vi "Trans-FPGA.vi"() -> ()   [LabVIEW 2016]
uses:
  Gate Valve Readback.ctl
  Faraday Cup Readback.ctl
  <vilib>/LabVIEW Targets/FPGA/cRIO/shared/nicrio_ModuleControls/nicrio_cRIO-9871_DataBitsEnum.ctl
  <vilib>/LabVIEW Targets/FPGA/cRIO/shared/nicrio_ModuleControls/nicrio_cRIO-9871_BaudRateEnum.ctl
  <vilib>/LabVIEW Targets/FPGA/cRIO/shared/nicrio_ModuleControls/nicrio_cRIO-9871_ParityEnum.ctl
  <vilib>/LabVIEW Targets/FPGA/cRIO/shared/nicrio_ModuleControls/nicrio_cRIO-9871_StopBitsEnum.ctl
  <vilib>/Platform/TimedLoop/XDataNode/timing_clust.ctl
  <vilib>/Platform/TimedLoop/XDataNode/nitl_modes.ctl
  <vilib>/Platform/TimedLoop/XDataNode/wakeup.ctl
  <vilib>/rvi/FXPMathLib/basic elements/FxpIntAccumulator/subVIs/nifxpmath_IntAccumulator_SimConfig.ctl
  <vilib>/rvi/Emulation/niFpgaGetClockAttributes.vi
  <vilib>/rvi/Emulation/niFpgaSctlEmulationGetInTimedLoop.vi
  <vilib>/rvi/Emulation/niFpgaEmulationReportErrorSimple.vi
  <vilib>/rvi/eio/common/nirviEmuTemplateMethod_errors.vi
  <vilib>/rvi/Emulation/niFpgaCriticalErrorInLSC.vi
  <vilib>/rvi/Analysis/common/codeGenErrors/XNode/niFpgaXNodeCodeGenErrorHandle.vi
  <vilib>/rvi/FXPMathLib/basic elements/FxpIntAccumulator/simVIs/DllFxpIntAccumulator_sub.vi
  <vilib>/rvi/eio/common/nirviEmuTemplatePropertySet_errors.vi
  <vilib>/eio/EIONode/EIONode.xnode
  <vilib>/rvi/Analysis/measure/dc-rms/XNode/niFpgaDC-RMS.xnode
  <vilib>/Platform/TimedLoop/XDataNode/XDataNode.xnode
  <vilib>/rvi/FXPMathLib/basic elements/FxpIntAccumulator/XNode/nifxpmath_IntAccumulator.xnode
  <vilib>/rvi/FXPMathLib/FxpMul/XNode/nifxpmath_Multiplier.xnode
  <vilib>/eio/EIOPropertyNode/EIOPropertyNode.xnode
  <vilib>/eio/EIOMethodNode/EIOMethodNode.xnode
  <vilib>/Platform/TimedLoop/XDataNode/XDNodeRunTimeDep.lvlib
  <vilib>/rvi/FXPMathLib/sim/FxpSim.dll
  <vilib>/rvi/eio/common/nirviEmuTemplatePropertyGet_errors.vi
  <vilib>/rvi/eio/common/nirviEmuTemplatePropertyGet_noerrors.vi
  <vilib>/rvi/eio/common/nirviEmuTemplatePropertySet_noerrors.vi
panel:
  in  "Analzyer Image FC Actuator":bool
  out "Analzyer Image FC Position":T1
  in  "Switch Object Interlock Bypass":bool
  in  "Analyzer Image Interlock Bypass":bool
  in  "Turbo 1 GV Actuator":bool
  in  "Beamline GV Actuator":bool
  in  "Turbo 2 GV Actuator":bool
  out "Analyzer Image Vac Interlock":bool
  out "Switch Object Vac Interlock":bool
  out "GV Interlock loop error":errorcluster
  out "Turbo 1 GV Status":T2
  out "Turbo 2 GV Status":T2
  out "Beamline GV Status":T2
  out "Actuator-Sensor Loop error":errorcluster
  in  "HV Enable":bool[](array[boolean])=[FALSE, FALSE, FALSE, FALSE, FALSE, FALSE]
  out "Switch Object Vacuum Error":errorcluster
  out "Analyze Image Vacuum Error":errorcluster
  out "Switch PS error":errorcluster
  out "ExB PS error":errorcluster
  out "Analyzer PS error":errorcluster
  out "9264 error":errorcluster
  out "9205 error":errorcluster
  in  "RT error":bool
  in  "switch mag ps set":u8[](array[numeric])=[0, 0, 0, 0, 0, 0, 0, 0, 0, 0]
  out "Switch mag data":u8
  out "Switch Mag Hall Probe Timed out":bool
  out "switch mag field":u8[](array[numeric])
  out "Switch Hall Probe error":errorcluster
  in  "trans ExB mag ps set":u8[](array[numeric])=[0, 0, 0, 0, 0, 0, 0, 0, 0, 0]
  in  "analyzer mag ps set":u8[](array[numeric])=[0, 0, 0, 0, 0, 0, 0, 0, 0, 0]
  out "analyzer mag data":u8
  out "Timed Out":bool
  out "analyzer mag field":u8[](array[numeric])
  out "Analyzer Hall Probe error":errorcluster
  out "Ion gauge 4":u8[](array[numeric])
  out "Convectron 4":u8[](array[numeric])
  out "Convectron 3":u8[](array[numeric])
  out "Ion gauge 3":u8[](array[numeric])
  out "Ion gauge 2":u8[](array[numeric])
  out "Convectron 2":u8[](array[numeric])
  out "Convectron 1":u8[](array[numeric])
  out "Ion gauge 1":u8[](array[numeric])
  in  "HV Set":fxp<+/-,26,5>[](array[numeric])=[0.0, 0.0, 0.0, 0.0, 0.0, 0.0] format="%.23g"
  out "HV monitor":fxp<+/-,26,5>[](array[numeric]) format="%.23g"
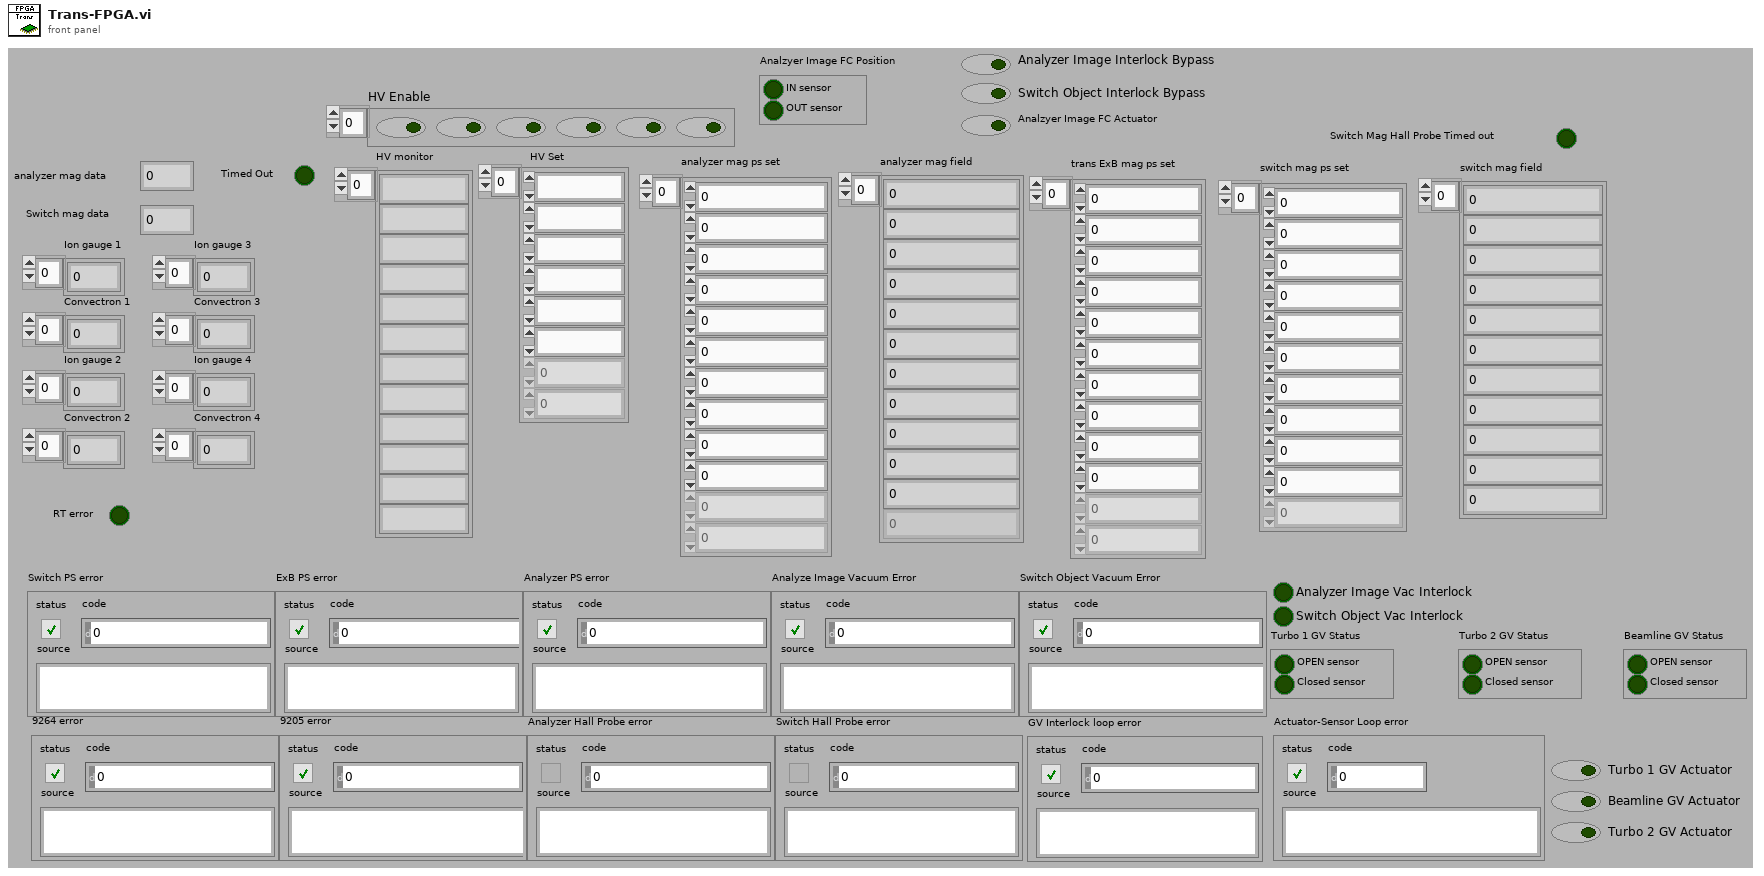
[diagram p1: front panel]
types:
  T1 = typedef "Faraday Cup Readback.ctl" = cluster{"IN sensor":bool, "OUT sensor":bool}
  T2 = typedef "Gate Valve Readback.ctl" = cluster{"OPEN sensor":bool, "Closed sensor":bool}
  T3 = typedef "nicrio_cRIO-9871_BaudRateEnum.ctl" = enum16{"75 bps", "110 bps", "134 bps", "150 bps", "300 bps", "600 bps", "1200 bps", "1800 bps", "2400 bps", "4800 bps", "7200 bps", "9600 bps", "14.4 kbps", "19.2 kbps", "28.8 kbps", "38.4 kbps", "57.6 kbps", "115.2 kbps", "230.4 kbps", "460.8 kbps", "921.6 kbps"}
  T4 = typedef "nicrio_cRIO-9871_DataBitsEnum.ctl" = enum8{"5", "6", "7", "8"}
  T5 = typedef "nicrio_cRIO-9871_StopBitsEnum.ctl" = enum8{"1", "1.5", "2"}
  T6 = typedef "nicrio_cRIO-9871_ParityEnum.ctl" = enum8{"None", "Odd", "Even", "Mark", "Space"}
  T7 = typedef "XDNodeRunTimeDep.lvlib/timing_clust.ctl" = cluster{"Expected End [f-1]":u64, "Actual End [f-1]":u64, "Finished Late? [f-1]":bool, "Expected End [i-1]":u64, "Actual End [i-1]":u64, "Finished Late? [i-1]":bool, "Expected Start [i]":u64, "Actual Start [i]":u64, "Expected Start [f]":u64, "Actual Start [f]":u64, "Source Name":string, "Structure Name":string, "Period":i64, "Deadline":i64, "Offset":i64, "Start":i64, "Priority":i32, "Timeout":i32, "Mode":T8, "Wakeup Reason":T9, "Error":errorcluster, "Source Type":string, "Secondary Source Type":string, "Global End Time":u64, "Global Start Time":u64, "Frame Duration":u64, "Iteration Duration":u64, "Assigned CPU":i32, "I/O Scan Engine Mode":u32}
  T8 = typedef "XDNodeRunTimeDep.lvlib/nitl_modes.ctl" = enum32{"No Change", "Process missed periods, maintain original phase", "Discard missed periods, maintain original phase", "Process missed periods, ignore original phase", "Discard missed periods, ignore original phase"}
  T9 = typedef "XDNodeRunTimeDep.lvlib/wakeup.ctl" = enum32{"Normal", "Aborted", "Asynchronous wakeup", "Timing source error", "Timed loop error", "Timeout"}
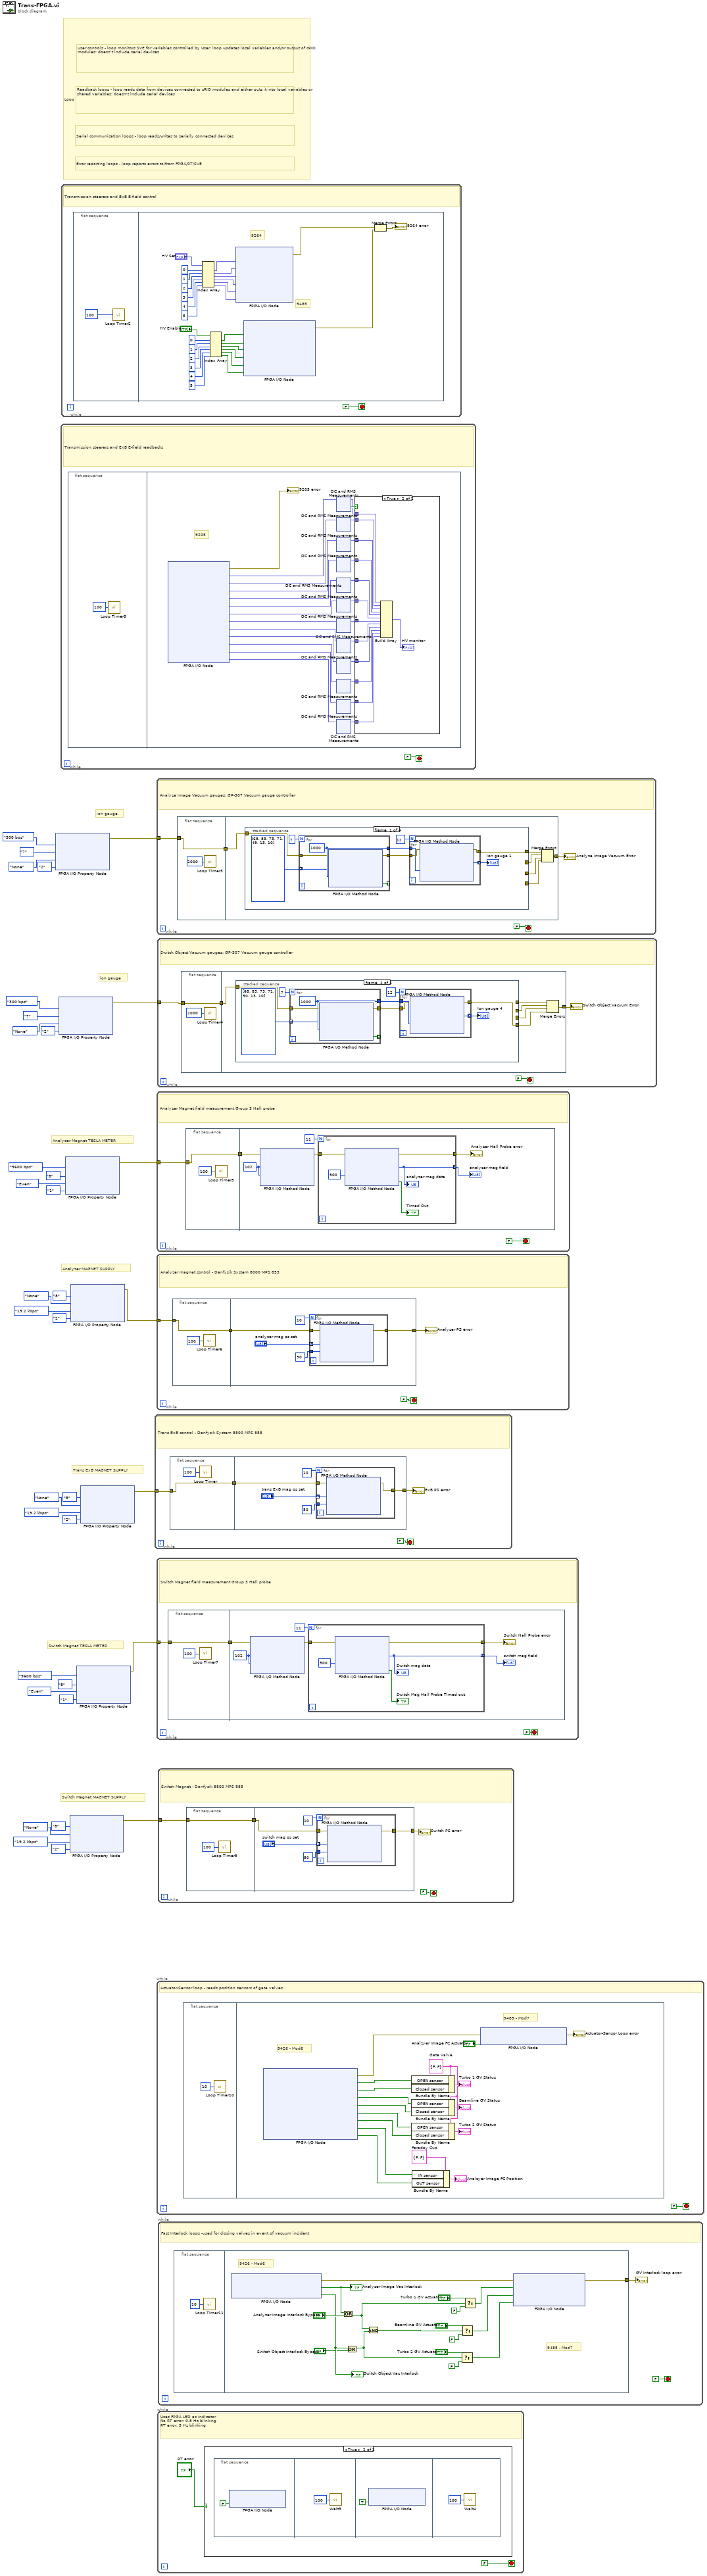
[diagram p0: block diagram]
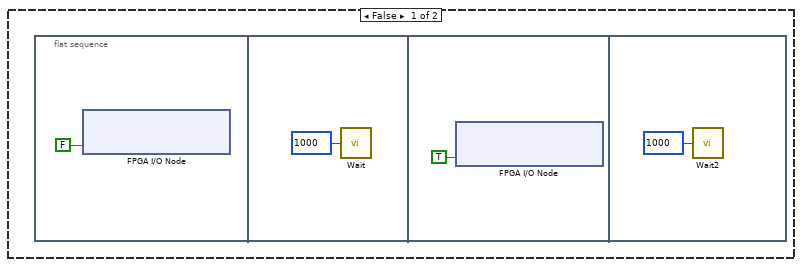
[diagram p2: hidden frame]
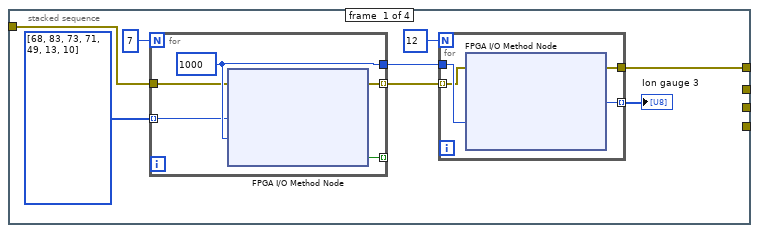
[diagram p4: hidden frame]
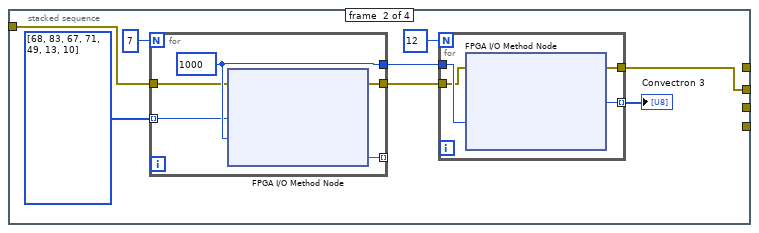
[diagram p5: hidden frame]
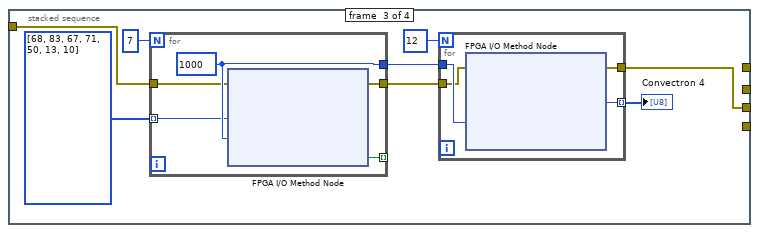
[diagram p6: hidden frame]
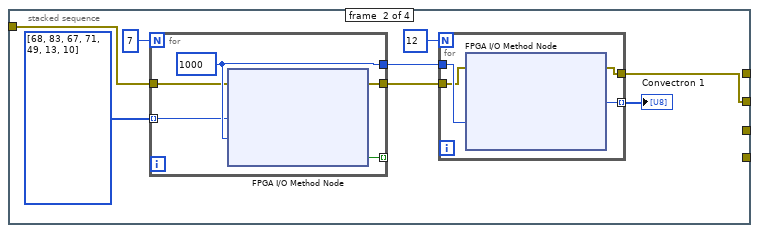
[diagram p7: hidden frame]
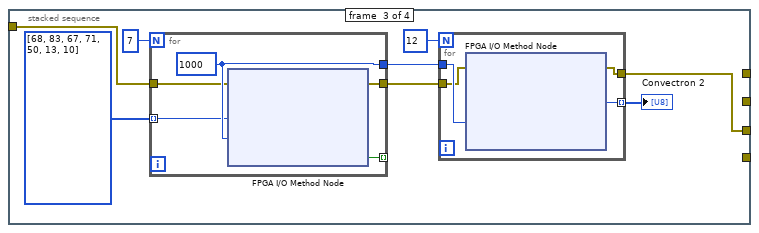
[diagram p8: hidden frame]
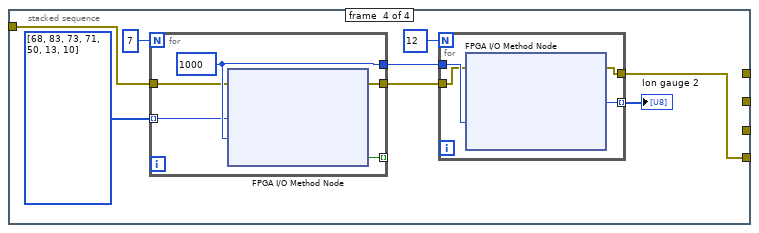
[diagram p9: hidden frame]
diagram:
  # "Error reporting loops - loop reports errors to/from FPGA/RT/SVE"
  # "Serial communication loops - loop reads/writes to serially connected devices"
  # "Readback loops - loop reads data from devices connected to cRIO modules and either puts it into local variables or shared variables; doesn't include serial devices"
  # "User controls - loop monitors SVE for variables controlled by User; loop updates local variables and/or output of cRIO modules; doesn't include serial devices"
  # "Loop legend - loops are color coded by responsibility"
  # "Switch Magnet TESLA METER"
  # "Switch Magnet MAGNET SUPPLY"
  # "Trans ExB MAGNET SUPPLY"
  # "ion gauge"
  # "Analyzer MAGNET SUPPLY"
  # "Analyzer Magnet TESLA METER"
  # "ion gauge"
  n1 = xnode "FPGA I/O Property Node"("Baud Rate"=nicrio_cRIO-9871_BaudRateEnum."300 bps", "Data Bits"=nicrio_cRIO-9871_DataBitsEnum."7", "Parity"=nicrio_cRIO-9871_ParityEnum."None", "Stop Bits"=nicrio_cRIO-9871_StopBitsEnum."2") -> ("error out"=w6:errorcluster)  [unwired: 2 in, 1 out]
  n2 = xnode "FPGA I/O Property Node"("Baud Rate"=nicrio_cRIO-9871_BaudRateEnum."300 bps", "Data Bits"=nicrio_cRIO-9871_DataBitsEnum."7", "Parity"=nicrio_cRIO-9871_ParityEnum."None", "Stop Bits"=nicrio_cRIO-9871_StopBitsEnum."2") -> ("error out"=w7:errorcluster)  [unwired: 2 in, 1 out]
  n3 = while {
    stop <- FALSE stop-if-true
    # "Transmission steerers and ExB E-field readbacks"
    n4 = flat-sequence {
      frame #0 {
        n5 = call "Loop Timer8"("Count(mSec)"=u32 100 ("Count(Ticks)")) -> ()  [unwired: 1 out]
      }
      frame #1 {
        # "9205"
        n6 = xnode "FPGA I/O Node"() -> ("error out"=→"9205 error":errorcluster, "X-steerer+ V read"=w62:fxp<+/-,26,5>, "X-steerer+ I read"=w60:fxp<+/-,26,5>, "X-steerer- V read"=w58:fxp<+/-,26,5>, "X-steerer- I read"=w56:fxp<+/-,26,5>, "Y-steerer+ V read"=w54:fxp<+/-,26,5>, "Y-steerer+ I read"=w52:fxp<+/-,26,5>, "Y-steerer- V read"=w50:fxp<+/-,26,5>, "Y-steerer- I read"=w48:fxp<+/-,26,5>, "ExB+ V read"=w46:fxp<+/-,26,5>, "ExB+ I read"=w44:fxp<+/-,26,5>, "ExB- V read"=w42:fxp<+/-,26,5>, "ExB- I read"=w40:fxp<+/-,26,5>)  [unwired: 13 in, 12 out]
        n7 = xnode "DC and RMS Measurements"("input data"=w62) -> ("DC"=w61:fxp<+/-,26,5>, "output valid"=w63:bool)  [unwired: 1 in]
        n8 = xnode "DC and RMS Measurements"("input data"=w60) -> ("DC"=w59:fxp<+/-,26,5>)  [unwired: 1 in, 1 out]
        n9 = xnode "DC and RMS Measurements"("input data"=w58) -> ("DC"=w57:fxp<+/-,26,5>)  [unwired: 1 in, 1 out]
        n10 = xnode "DC and RMS Measurements"("input data"=w56) -> ("DC"=w55:fxp<+/-,26,5>)  [unwired: 1 in, 1 out]
        n11 = xnode "DC and RMS Measurements"("input data"=w54) -> ("DC"=w53:fxp<+/-,26,5>)  [unwired: 1 in, 1 out]
        n12 = xnode "DC and RMS Measurements"("input data"=w52) -> ("DC"=w51:fxp<+/-,26,5>)  [unwired: 1 in, 1 out]
        n13 = xnode "DC and RMS Measurements"("input data"=w50) -> ("DC"=w49:fxp<+/-,26,5>)  [unwired: 1 in, 1 out]
        n14 = xnode "DC and RMS Measurements"("input data"=w48) -> ("DC"=w47:fxp<+/-,26,5>)  [unwired: 1 in, 1 out]
        n15 = xnode "DC and RMS Measurements"("input data"=w46) -> ("DC"=w45:fxp<+/-,26,5>)  [unwired: 1 in, 1 out]
        n16 = xnode "DC and RMS Measurements"("input data"=w44) -> ("DC"=w43:fxp<+/-,26,5>)  [unwired: 1 in, 1 out]
        n17 = xnode "DC and RMS Measurements"("input data"=w42) -> ("DC"=w41:fxp<+/-,26,5>)  [unwired: 1 in, 1 out]
        n18 = xnode "DC and RMS Measurements"("input data"=w40) -> ("DC"=w39:fxp<+/-,26,5>)  [unwired: 1 in, 1 out]
        n19 = case shown="True" w63 {
          tunnel: w61 -> [_ w76]
          tunnel: w59 -> [_ w75]
          tunnel: w57 -> [_ w74]
          tunnel: w55 -> [_ w73]
          tunnel: w53 -> [_ w72]
          tunnel: w51 -> [_ w71]
          tunnel: w49 -> [_ w70]
          tunnel: w47 -> [_ w69]
          tunnel: w45 -> [_ w68]
          tunnel: w43 -> [_ w67]
          tunnel: w41 -> [_ w66]
          tunnel: w39 -> [_ w65]
          frame False {
          }
          frame True {
            n20 = Build Array(w76, w75, w74, w73, w72, w71, w70, w69, w68, w67, w66, w65) -> (→"HV monitor":fxp<+/-,26,5>[])
          }
        }
      }
    }
  }
  n21 = while {
    stop <- FALSE stop-if-true
    # "Transmission steerers and ExB E-field control"
    n22 = flat-sequence {
      frame #0 {
        n23 = call "Loop Timer2"("Count(mSec)"=u32 100 ("Count(Ticks)")) -> ()  [unwired: 1 out]
      }
      frame #1 {
        # "9485"
        # "9264"
        n24 = Index Array(array="HV Set", index #1=0 ("index"), index #2=1 ("index"), index #3=2 ("index"), index #4=3 ("index"), index #5=4 ("index"), index #6=5 ("index")) -> (element #1=w1062:fxp<+/-,26,5>, element #2=w1061:fxp<+/-,26,5>, element #3=w1060:fxp<+/-,26,5>, element #4=w1055:fxp<+/-,26,5>, element #5=w1057:fxp<+/-,26,5>, element #6=w1056:fxp<+/-,26,5>)
        n25 = Index Array(array="HV Enable", index #1=0 ("index"), index #2=1 ("index"), index #3=2 ("index"), index #4=3 ("index"), index #5=4 ("index"), index #6=5 ("index")) -> (element #1=w1045:bool, element #2=w1044:bool, element #3=w1043:bool, element #4=w1042:bool, element #5=w1041:bool, element #6=w1040:bool)
        n26 = xnode "FPGA I/O Node"("X-steerer+ V set"=w1062, "X-steerer- V set"=w1061, "Y-steerer+ V set"=w1060, "Y-steerer- V set"=w1055, "ExB+ V set"=w1057, "ExB- V set"=w1056) -> ("error out"=w1054:errorcluster)  [unwired: 7 in, 6 out]
        n27 = xnode "FPGA I/O Node"("X-Steerer+ HV Enable"=w1045, "X-Steerer- HV Enable"=w1044, "Y-Steerer+ HV Enable"=w1043, "Y-Steerer- HV Enable"=w1042, "ExB+ HV Enable"=w1041, "ExB- HV Enable"=w1040) -> ("error out"=w1052:errorcluster)  [unwired: 7 in, 6 out]
        n28 = Merge Errors(w1054, w1052) -> (→"9264 error":errorcluster)
      }
    }
  }
  n29 = xnode "FPGA I/O Property Node"("Baud Rate"=nicrio_cRIO-9871_BaudRateEnum."9600 bps", "Data Bits"=nicrio_cRIO-9871_DataBitsEnum."8", "Parity"=nicrio_cRIO-9871_ParityEnum."Even", "Stop Bits"=nicrio_cRIO-9871_StopBitsEnum."1") -> ("error out"=w8:errorcluster)  [unwired: 2 in, 1 out]
  n30 = xnode "FPGA I/O Property Node"("Data Bits"=nicrio_cRIO-9871_DataBitsEnum."8", "Parity"=nicrio_cRIO-9871_ParityEnum."None", "Baud Rate"=nicrio_cRIO-9871_BaudRateEnum."19.2 kbps", "Stop Bits"=nicrio_cRIO-9871_StopBitsEnum."2") -> ("error out"=w10:errorcluster)  [unwired: 2 in, 1 out]
  n31 = xnode "FPGA I/O Property Node"("Data Bits"=nicrio_cRIO-9871_DataBitsEnum."8", "Parity"=nicrio_cRIO-9871_ParityEnum."None", "Baud Rate"=nicrio_cRIO-9871_BaudRateEnum."19.2 kbps", "Stop Bits"=nicrio_cRIO-9871_StopBitsEnum."2") -> ("error out"=w9:errorcluster)  [unwired: 2 in, 1 out]
  n32 = xnode "FPGA I/O Property Node"("Baud Rate"=nicrio_cRIO-9871_BaudRateEnum."9600 bps", "Data Bits"=nicrio_cRIO-9871_DataBitsEnum."8", "Parity"=nicrio_cRIO-9871_ParityEnum."Even", "Stop Bits"=nicrio_cRIO-9871_StopBitsEnum."1") -> ("error out"=w11:errorcluster)  [unwired: 2 in, 1 out]
  n33 = xnode "FPGA I/O Property Node"("Data Bits"=nicrio_cRIO-9871_DataBitsEnum."8", "Parity"=nicrio_cRIO-9871_ParityEnum."None", "Baud Rate"=nicrio_cRIO-9871_BaudRateEnum."19.2 kbps", "Stop Bits"=nicrio_cRIO-9871_StopBitsEnum."2") -> ("error out"=w12:errorcluster)  [unwired: 2 in, 1 out]
  n34 = while {
    tunnel: w12 -> [w1069]
    stop <- FALSE stop-if-true
    # "Trans ExB control - Danfysik System 8500 MPS 858"
    n35 = flat-sequence {
      tunnel: w1069 -> [w1072]
      tunnel: [w1072] -> w1068
      tunnel: [w1075] -> w1070
      tunnel: w1068 -> [w1074]
      frame #0 {
        n36 = call "Loop Timer"("Count(mSec)"=u32 100) -> ()  [unwired: 1 out]
      }
      frame #1 {
        n37 = for {
          N: 10 -> [_]
          tunnel: 50 ("Timeout (ms)") -> [w1082]
          tunnel: "trans ExB mag ps set" -> [w1081] mode=indexing
          tunnel: [w1080] -> w1075
          tunnel: w1074 -> [w1079]
          n38 = xnode "FPGA I/O Method Node"("error in"=w1079, "Data"=w1081, "Timeout (ms)"=w1082) -> ("error out"=w1080:errorcluster)  [unwired: 1 in, 2 out]
        }
      }
    }
    "ExB PS error" <- w1070
  }
  n39 = while {
    tunnel: w6 -> [w1085]
    stop <- FALSE stop-if-true
    # "Analyze Image Vacuum gauges: GP-307 Vacuum gauge controller"
    n40 = flat-sequence {
      tunnel: w1085 -> [w1087]
      tunnel: [w1087] -> w1084
      tunnel: w1084 -> [w1094]
      tunnel: [w1092] -> w1083
      frame #0 {
        n41 = call "Loop Timer3"("Count(mSec)"=u32 2000 ("Count(Ticks)")) -> ()  [unwired: 1 out]
      }
      frame #1 {
        n42 = stacked-sequence {
          tunnel: w1094 -> [w1097 w1114 w1131 w1147]
          tunnel: [w1095 _ _ _] -> w1093
          tunnel: [_ w1112 _ _] -> w1091
          tunnel: [_ _ w1129 _] -> w1090
          tunnel: [_ _ _ w1146] -> w1089
          frame #0 {
            n43 = for {
              N: 7 -> [_]
              tunnel: [w1111] -> w1102
              tunnel: [w1110] -> _ mode=indexing
              tunnel: u8[] [68, 83, 73, 71, 49, 13, 10] ("unsigned byte array") -> [w1109] mode=indexing
              tunnel: w1097 -> [w1108]
              tunnel: [w1107] -> w1096
              w1111 = 1000 ("Timeout (ms)")
              n44 = xnode "FPGA I/O Method Node"("error in"=w1108, "Data"=w1109, "Timeout (ms)"=w1111) -> ("error out"=w1107:errorcluster, "Timed Out"=w1110:bool)  [unwired: 1 in, 1 out]
            }
            n45 = for {
              N: 12 -> [_]
              tunnel: w1102 -> [w1106]
              tunnel: [w1105] -> w1098 mode=indexing
              tunnel: w1096 -> [w1104]
              tunnel: [w1103] -> w1095
              n46 = xnode "FPGA I/O Method Node"("error in"=w1104, "Timeout (ms)"=w1106) -> ("error out"=w1103:errorcluster, "Data"=w1105:u8)  [unwired: 1 in, 2 out]
            }
            "Ion gauge 1" <- w1098
          }
          frame #1 {
            n47 = for {
              N: 7 -> [_]
              tunnel: [w1128] -> w1119
              tunnel: [w1127] -> _ mode=indexing
              tunnel: u8[] [68, 83, 67, 71, 49, 13, 10] ("unsigned byte array") -> [w1126] mode=indexing
              tunnel: w1114 -> [w1125]
              tunnel: [w1124] -> w1113
              w1128 = 1000 ("Timeout (ms)")
              n48 = xnode "FPGA I/O Method Node"("error in"=w1125, "Data"=w1126, "Timeout (ms)"=w1128) -> ("error out"=w1124:errorcluster, "Timed Out"=w1127:bool)  [unwired: 1 in, 1 out]
            }
            n49 = for {
              N: 12 -> [_]
              tunnel: w1119 -> [w1123]
              tunnel: [w1122] -> w1115 mode=indexing
              tunnel: w1113 -> [w1121]
              tunnel: [w1120] -> w1112
              n50 = xnode "FPGA I/O Method Node"("error in"=w1121, "Timeout (ms)"=w1123) -> ("error out"=w1120:errorcluster, "Data"=w1122:u8)  [unwired: 1 in, 2 out]
            }
            "Convectron 1" <- w1115
          }
          frame #2 {
            n51 = for {
              N: 7 -> [_]
              tunnel: [w1145] -> w1136
              tunnel: [w1144] -> _ mode=indexing
              tunnel: u8[] [68, 83, 67, 71, 50, 13, 10] ("unsigned byte array") -> [w1143] mode=indexing
              tunnel: w1131 -> [w1142]
              tunnel: [w1141] -> w1130
              w1145 = 1000 ("Timeout (ms)")
              n52 = xnode "FPGA I/O Method Node"("error in"=w1142, "Data"=w1143, "Timeout (ms)"=w1145) -> ("error out"=w1141:errorcluster, "Timed Out"=w1144:bool)  [unwired: 1 in, 1 out]
            }
            n53 = for {
              N: 12 -> [_]
              tunnel: w1136 -> [w1140]
              tunnel: [w1139] -> w1132 mode=indexing
              tunnel: w1130 -> [w1138]
              tunnel: [w1137] -> w1129
              n54 = xnode "FPGA I/O Method Node"("error in"=w1138, "Timeout (ms)"=w1140) -> ("error out"=w1137:errorcluster, "Data"=w1139:u8)  [unwired: 1 in, 2 out]
            }
            "Convectron 2" <- w1132
          }
          frame #3 {
            n55 = for {
              N: 7 -> [_]
              tunnel: [w1162] -> w1153
              tunnel: [w1161] -> _ mode=indexing
              tunnel: u8[] [68, 83, 73, 71, 50, 13, 10] ("unsigned byte array") -> [w1160] mode=indexing
              tunnel: [w1159] -> w1148
              tunnel: w1147 -> [w1158]
              w1162 = 1000 ("Timeout (ms)")
              n56 = xnode "FPGA I/O Method Node"("error in"=w1158, "Data"=w1160, "Timeout (ms)"=w1162) -> ("error out"=w1159:errorcluster, "Timed Out"=w1161:bool)  [unwired: 1 in, 1 out]
            }
            n57 = for {
              N: 12 -> [_]
              tunnel: w1153 -> [w1157]
              tunnel: [w1156] -> w1149 mode=indexing
              tunnel: w1148 -> [w1155]
              tunnel: [w1154] -> w1146
              n58 = xnode "FPGA I/O Method Node"("error in"=w1155, "Timeout (ms)"=w1157) -> ("error out"=w1154:errorcluster, "Data"=w1156:u8)  [unwired: 1 in, 2 out]
            }
            "Ion gauge 2" <- w1149
          }
        }
        n59 = Merge Errors(w1093, w1091, w1090, w1089) -> (w1092:errorcluster)
      }
    }
    "Analyze Image Vacuum Error" <- w1083
  }
  n60 = while {
    tunnel: w8 -> [w1164]
    stop <- FALSE stop-if-true
    # "Analyzer Magnet field measurement Group 3 Hall probe"
    n61 = flat-sequence {
      tunnel: w1164 -> [w1166]
      tunnel: [w1166] -> w1163
      tunnel: w1163 -> [w1168]
      frame #0 {
        n62 = call "Loop Timer5"("Count(mSec)"=u32 100) -> ()  [unwired: 1 out]
      }
      frame #1 {
        w1172 = u8 102 ("Data")
        n63 = xnode "FPGA I/O Method Node"("error in"=w1168, "Data"=w1172, "Timeout (ms)"=w1172) -> ("error out"=w1171:errorcluster)  [unwired: 1 in, 2 out]
        n64 = for {
          N: 11 ("Numeric 3") -> [_]
          tunnel: [w1176] -> w1169 mode=indexing
          tunnel: w1171 -> [w1175]
          tunnel: [w1174] -> w1170
          n65 = xnode "FPGA I/O Method Node"("error in"=w1175, "Timeout (ms)"=500) -> ("error out"=w1174:errorcluster, "Data"=w1176:u8, "Timed Out"=→"Timed Out":bool)  [unwired: 1 in, 1 out]
          "analyzer mag data" <- w1176
        }
        "analyzer mag field" <- w1169
        "Analyzer Hall Probe error" <- w1170
      }
    }
  }
  n66 = while {
    tunnel: w9 -> [w1180]
    stop <- FALSE stop-if-true
    # "Analyzer magnet control - Danfysik System 8000 MPS 853"
    n67 = flat-sequence {
      tunnel: w1180 -> [w1183]
      tunnel: [w1183] -> w1179
      tunnel: [w1186] -> w1181
      tunnel: w1179 -> [w1185]
      frame #0 {
        n68 = call "Loop Timer6"("Count(mSec)"=u32 100) -> ()  [unwired: 1 out]
      }
      frame #1 {
        n69 = for {
          N: 10 -> [_]
          tunnel: 50 ("Timeout (ms)") -> [w1193]
          tunnel: "analyzer mag ps set" -> [w1192] mode=indexing
          tunnel: [w1191] -> w1186
          tunnel: w1185 -> [w1190]
          n70 = xnode "FPGA I/O Method Node"("error in"=w1190, "Data"=w1192, "Timeout (ms)"=w1193) -> ("error out"=w1191:errorcluster)  [unwired: 1 in, 2 out]
        }
      }
    }
    "Analyzer PS error" <- w1181
  }
  n71 = while {
    tunnel: w11 -> [w1195]
    stop <- FALSE stop-if-true
    # "Switch Magnet field measurement Group 3 Hall probe"
    n72 = flat-sequence {
      tunnel: w1195 -> [w1197]
      tunnel: [w1197] -> w1194
      tunnel: w1194 -> [w1200]
      frame #0 {
        n73 = call "Loop Timer7"("Count(mSec)"=u32 100) -> ()  [unwired: 1 out]
      }
      frame #1 {
        w1203 = u8 102 ("Data")
        n74 = xnode "FPGA I/O Method Node"("error in"=w1200, "Data"=w1203, "Timeout (ms)"=w1203) -> ("error out"=w1202:errorcluster)  [unwired: 1 in, 2 out]
        n75 = for {
          N: 11 ("Numeric 3") -> [_]
          tunnel: [w1207] -> w1199 mode=indexing
          tunnel: w1202 -> [w1206]
          tunnel: [w1205] -> w1201
          n76 = xnode "FPGA I/O Method Node"("error in"=w1206, "Timeout (ms)"=500) -> ("error out"=w1205:errorcluster, "Data"=w1207:u8, "Timed Out"=→"Switch Mag Hall Probe Timed out":bool)  [unwired: 1 in, 1 out]
          "Switch mag data" <- w1207
        }
        "switch mag field" <- w1199
        "Switch Hall Probe error" <- w1201
      }
    }
  }
  n77 = while {
    stop <- FALSE stop-if-true
    # "Actuator-Sensor loop - reads position sensors of gate valves"
    n78 = flat-sequence {
      frame #0 {
        n79 = call "Loop Timer10"("Count(uSec)"=u32 10) -> ()  [unwired: 1 out]
      }
      frame #1 {
        w1218 = T1 {"IN sensor"=FALSE, "OUT sensor"=FALSE}  # Faraday Cup
        w1227 = T2 {"OPEN sensor"=FALSE, "Closed sensor"=FALSE}  # Gate Valve
        # "9485 - Mod7"
        # "9426 - Mod6"
        n80 = xnode "FPGA I/O Node"() -> ("error out"=w1213:errorcluster, "Turbo 1 GV OPEN sensor"=w1226:bool, "Turbo 1 GV CLOSED sensor"=w1225:bool, "Beamline GV OPEN sensor"=w1224:bool, "Beamline GV CLOSED sensor"=w1223:bool, "Turbo 2 GV OPEN sensor"=w1220:bool, "Turbo 2 GV CLOSED sensor"=w1219:bool, "Analyzer Image FC IN sensor"=w1216:bool, "Analyzer Image FC OUT sensor"=w1215:bool)  [unwired: 9 in, 8 out]
        n81 = Bundle By Name(cluster=w1227, "OPEN sensor"=w1226, "Closed sensor"=w1225) -> (→"Turbo 1 GV Status":T2)
        n82 = Bundle By Name(cluster=w1227, "OPEN sensor"=w1224, "Closed sensor"=w1223) -> (→"Beamline GV Status":T2)
        n83 = Bundle By Name(cluster=w1227, "OPEN sensor"=w1220, "Closed sensor"=w1219) -> (→"Turbo 2 GV Status":T2)
        n84 = Bundle By Name(cluster=w1218, "IN sensor"=w1216, "OUT sensor"=w1215) -> (→"Analzyer Image FC Position":T1)
        n85 = xnode "FPGA I/O Node"("error in"=w1213, "Analyzer Image FC actuator"="Analzyer Image FC Actuator") -> ("error out"=→"Actuator-Sensor Loop error":errorcluster)  [unwired: 1 in, 1 out]
      }
    }
  }
  n86 = while {
    tunnel: w7 -> [w1231]
    stop <- FALSE stop-if-true
    # "Switch Object Vacuum gauges: GP-307 Vacuum gauge controller"
    n87 = flat-sequence {
      tunnel: w1231 -> [w1233]
      tunnel: [w1233] -> w1230
      tunnel: w1230 -> [w1240]
      tunnel: [w1238] -> w1229
      frame #0 {
        n88 = call "Loop Timer4"("Count(mSec)"=u32 2000 ("Count(Ticks)")) -> ()  [unwired: 1 out]
      }
      frame #1 {
        n89 = stacked-sequence {
          tunnel: w1240 -> [w1243 w1260 w1277 w1294]
          tunnel: [w1241 _ _ _] -> w1239
          tunnel: [_ w1258 _ _] -> w1237
          tunnel: [_ _ w1275 _] -> w1236
          tunnel: [_ _ _ w1292] -> w1235
          frame #0 {
            n90 = for {
              N: 7 -> [_]
              tunnel: [w1257] -> w1248
              tunnel: [w1256] -> _ mode=indexing
              tunnel: u8[] [68, 83, 73, 71, 49, 13, 10] ("unsigned byte array") -> [w1255] mode=indexing
              tunnel: w1243 -> [w1254]
              tunnel: [w1253] -> w1242 mode=indexing
              w1257 = 1000 ("Timeout (ms)")
              n91 = xnode "FPGA I/O Method Node"("error in"=w1254, "Data"=w1255, "Timeout (ms)"=w1257) -> ("error out"=w1253:errorcluster, "Timed Out"=w1256:bool)  [unwired: 1 in, 1 out]
            }
            n92 = for {
              N: 12 -> [_]
              tunnel: w1248 -> [w1252]
              tunnel: [w1251] -> w1244 mode=indexing
              tunnel: w1242 -> [w1250] mode=indexing
              tunnel: [w1249] -> w1241
              n93 = xnode "FPGA I/O Method Node"("error in"=w1250, "Timeout (ms)"=w1252) -> ("error out"=w1249:errorcluster, "Data"=w1251:u8)  [unwired: 1 in, 2 out]
            }
            "Ion gauge 3" <- w1244
          }
          frame #1 {
            n94 = for {
              N: 7 -> [_]
              tunnel: [w1274] -> w1265
              tunnel: [w1273] -> _ mode=indexing
              tunnel: u8[] [68, 83, 67, 71, 49, 13, 10] ("unsigned byte array") -> [w1272] mode=indexing
              tunnel: w1260 -> [w1271]
              tunnel: [w1270] -> w1259
              w1274 = 1000 ("Timeout (ms)")
              n95 = xnode "FPGA I/O Method Node"("error in"=w1271, "Data"=w1272, "Timeout (ms)"=w1274) -> ("error out"=w1270:errorcluster, "Timed Out"=w1273:bool)  [unwired: 1 in, 1 out]
            }
            n96 = for {
              N: 12 -> [_]
              tunnel: w1265 -> [w1269]
              tunnel: [w1268] -> w1261 mode=indexing
              tunnel: w1259 -> [w1267]
              tunnel: [w1266] -> w1258
              n97 = xnode "FPGA I/O Method Node"("error in"=w1267, "Timeout (ms)"=w1269) -> ("error out"=w1266:errorcluster, "Data"=w1268:u8)  [unwired: 1 in, 2 out]
            }
            "Convectron 3" <- w1261
          }
          frame #2 {
            n98 = for {
              N: 7 -> [_]
              tunnel: [w1291] -> w1282
              tunnel: [w1290] -> _ mode=indexing
              tunnel: u8[] [68, 83, 67, 71, 50, 13, 10] ("unsigned byte array") -> [w1289] mode=indexing
              tunnel: w1277 -> [w1288]
              tunnel: [w1287] -> w1276
              w1291 = 1000 ("Timeout (ms)")
              n99 = xnode "FPGA I/O Method Node"("error in"=w1288, "Data"=w1289, "Timeout (ms)"=w1291) -> ("error out"=w1287:errorcluster, "Timed Out"=w1290:bool)  [unwired: 1 in, 1 out]
            }
            n100 = for {
              N: 12 -> [_]
              tunnel: w1282 -> [w1286]
              tunnel: [w1285] -> w1278 mode=indexing
              tunnel: w1276 -> [w1284]
              tunnel: [w1283] -> w1275
              n101 = xnode "FPGA I/O Method Node"("error in"=w1284, "Timeout (ms)"=w1286) -> ("error out"=w1283:errorcluster, "Data"=w1285:u8)  [unwired: 1 in, 2 out]
            }
            "Convectron 4" <- w1278
          }
          frame #3 {
            n102 = for {
              N: 7 -> [_]
              tunnel: [w1308] -> w1299
              tunnel: [w1307] -> _ mode=indexing
              tunnel: u8[] [68, 83, 73, 71, 50, 13, 10] ("unsigned byte array") -> [w1306] mode=indexing
              tunnel: w1294 -> [w1305]
              tunnel: [w1304] -> w1293
              w1308 = 1000 ("Timeout (ms)")
              n103 = xnode "FPGA I/O Method Node"("error in"=w1305, "Data"=w1306, "Timeout (ms)"=w1308) -> ("error out"=w1304:errorcluster, "Timed Out"=w1307:bool)  [unwired: 1 in, 1 out]
            }
            n104 = for {
              N: 12 -> [_]
              tunnel: w1299 -> [w1303]
              tunnel: [w1302] -> w1295 mode=indexing
              tunnel: w1293 -> [w1301]
              tunnel: [w1300] -> w1292
              n105 = xnode "FPGA I/O Method Node"("error in"=w1301, "Timeout (ms)"=w1303) -> ("error out"=w1300:errorcluster, "Data"=w1302:u8)  [unwired: 1 in, 2 out]
            }
            "Ion gauge 4" <- w1295
          }
        }
        n106 = Merge Errors(w1239, w1237, w1236, w1235) -> (w1238:errorcluster)
      }
    }
    "Switch Object Vacuum Error" <- w1229
  }
  n107 = while {
    stop <- FALSE stop-if-true
    # "Uses FPGA LED as indicator\nNo RT error: 0.5 Hz blinking\nRT error: 5 Hz blinking"
    n108 = case shown="True" "RT error" {
      frame False {
        n109 = flat-sequence {
          frame #0 {
            n110 = xnode "FPGA I/O Node"("USER FPGA LED"=FALSE ("FPGA LED")) -> ()  [unwired: 1 in, 1 out]
          }
          frame #1 {
            n111 = call "Wait"("Count(mSec)"=u16 1000) -> ()  [unwired: 1 out]
          }
          frame #2 {
            n112 = xnode "FPGA I/O Node"("USER FPGA LED"=TRUE ("FPGA LED")) -> ()  [unwired: 1 in, 1 out]
          }
          frame #3 {
            n113 = call "Wait2"("Count(mSec)"=u16 1000) -> ()  [unwired: 1 out]
          }
        }
      }
      frame True {
        n114 = flat-sequence {
          frame #0 {
            n115 = xnode "FPGA I/O Node"("USER FPGA LED"=FALSE ("FPGA LED")) -> ()  [unwired: 1 in, 1 out]
          }
          frame #1 {
            n116 = call "Wait3"("Count(mSec)"=u16 100) -> ()  [unwired: 1 out]
          }
          frame #2 {
            n117 = xnode "FPGA I/O Node"("USER FPGA LED"=TRUE ("FPGA LED")) -> ()  [unwired: 1 in, 1 out]
          }
          frame #3 {
            n118 = call "Wait4"("Count(mSec)"=u16 100) -> ()  [unwired: 1 out]
          }
        }
      }
    }
  }
  n119 = while {
    tunnel: w10 -> [w1319]
    stop <- FALSE stop-if-true
    # "Switch Magnet - Danfysik 8800 MPS 883"
    n120 = flat-sequence {
      tunnel: [w1323] -> w1320
      tunnel: w1319 -> [w1323]
      tunnel: [w1326] -> w1321
      tunnel: w1320 -> [w1325]
      frame #0 {
        n121 = call "Loop Timer9"("Count(mSec)"=u32 100) -> ()  [unwired: 1 out]
      }
      frame #1 {
        n122 = for {
          N: 10 -> [_]
          tunnel: 50 ("Timeout (ms)") -> [w1333]
          tunnel: "switch mag ps set" -> [w1332] mode=indexing
          tunnel: [w1331] -> w1326
          tunnel: w1325 -> [w1330]
          n123 = xnode "FPGA I/O Method Node"("error in"=w1330, "Data"=w1332, "Timeout (ms)"=w1333) -> ("error out"=w1331:errorcluster)  [unwired: 1 in, 2 out]
        }
      }
    }
    "Switch PS error" <- w1321
  }
  n124 = while {
    stop <- FALSE stop-if-true
    # "Fast Interlock loops -used for closing valves in event of vacuum incident"
    n125 = flat-sequence {
      tunnel: [w1346] -> w1334
      frame #0 {
        n126 = call "Loop Timer11"("Count(uSec)"=u32 10) -> ()  [unwired: 1 out]
      }
      frame #1 {
        # "9485 - Mod7"
        # "9426 - Mod6"
        n127 = xnode "FPGA I/O Node"() -> ("error out"=w1354:errorcluster, "Analyzer Image Vac Interlock"=w1341:bool, "Switch Object Vac Interlock"=w1339:bool)  [unwired: 3 in, 2 out]
        "Analyzer Image Vac Interlock" <- w1341
        "Switch Object Vac Interlock" <- w1339
        n128 = Or(x=w1341, y="Analyzer Image Interlock Bypass") -> (x .or. y?=w1342:bool)
        n129 = Or(x=w1339, y="Switch Object Interlock Bypass") -> (x .or. y?=w1338:bool)
        n130 = And(x=w1342, y=w1338) -> (x .and. y?=w1349:bool)
        n131 = Select(t="Turbo 2 GV Actuator", s=w1338, f=FALSE) -> (s? t:f=w1343:bool)
        n132 = Select(t="Beamline GV Actuator", s=w1349, f=FALSE) -> (s? t:f=w1344:bool)
        n133 = Select(t="Turbo 1 GV Actuator", s=w1342, f=FALSE) -> (s? t:f=w1345:bool)
        n134 = xnode "FPGA I/O Node"("error in"=w1354, "Turbo 1 GV actuator"=w1345, "Beamline GV actuator"=w1344, "Turbo 2 GV actuator"=w1343) -> ("error out"=w1346:errorcluster)  [unwired: 3 in, 3 out]
      }
    }
    "GV Interlock loop error" <- w1334
  }
